vi "VSG25A_Main.vi"() -> ()   [LabVIEW 2014]
uses:
  Queue Control.ctl
  sg_lib/VSG25A.lvlib
panel:
  in  "RF On":bool
  in  "CW Button":bool
  in  "Sweep Button":bool
  in  "Ramp Button":bool
  in  "QAM Button":bool
  in  "FSK Button":bool
  in  "Multitone Button":bool
  in  "Pulse Button":bool
  in  "FM Button":bool
  in  "AM Button":bool
  in  "Amplitude (dBm)":dbl caption="Frequency"
  in  "Exit Button":bool caption="Blank Button"
  in  "Error In":errorcluster
  in  "Frequency":dbl
  in  "Connect Button":bool caption="Blank Button"
  out "Error Out":errorcluster
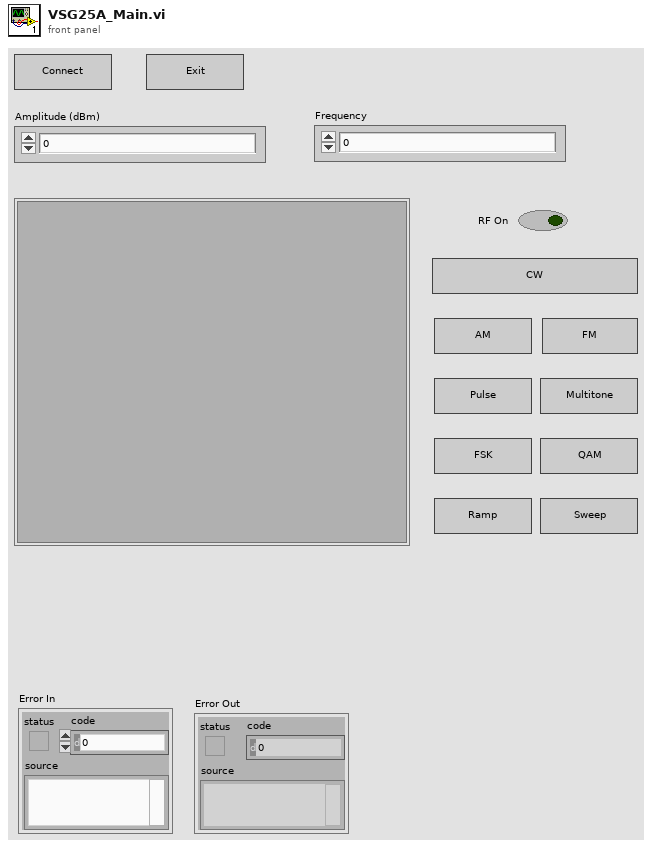
[diagram p1: front panel]
types:
  T1 = cluster{"Command":enum16{"Exit", "Connect"}, "Data":variant}
  T2 = typedef "Queue Control.ctl" = cluster{"Command":enum16{"Connect", "Exit", "RF On", "CW", "Sweep"}, "Data":variant}
  T3 = enum16{"Init", "Proc GUI Events", "Dispatch", "Exit"}
  T4 = enum16{"Connect", "Exit", "RF On", "CW", "Sweep"}
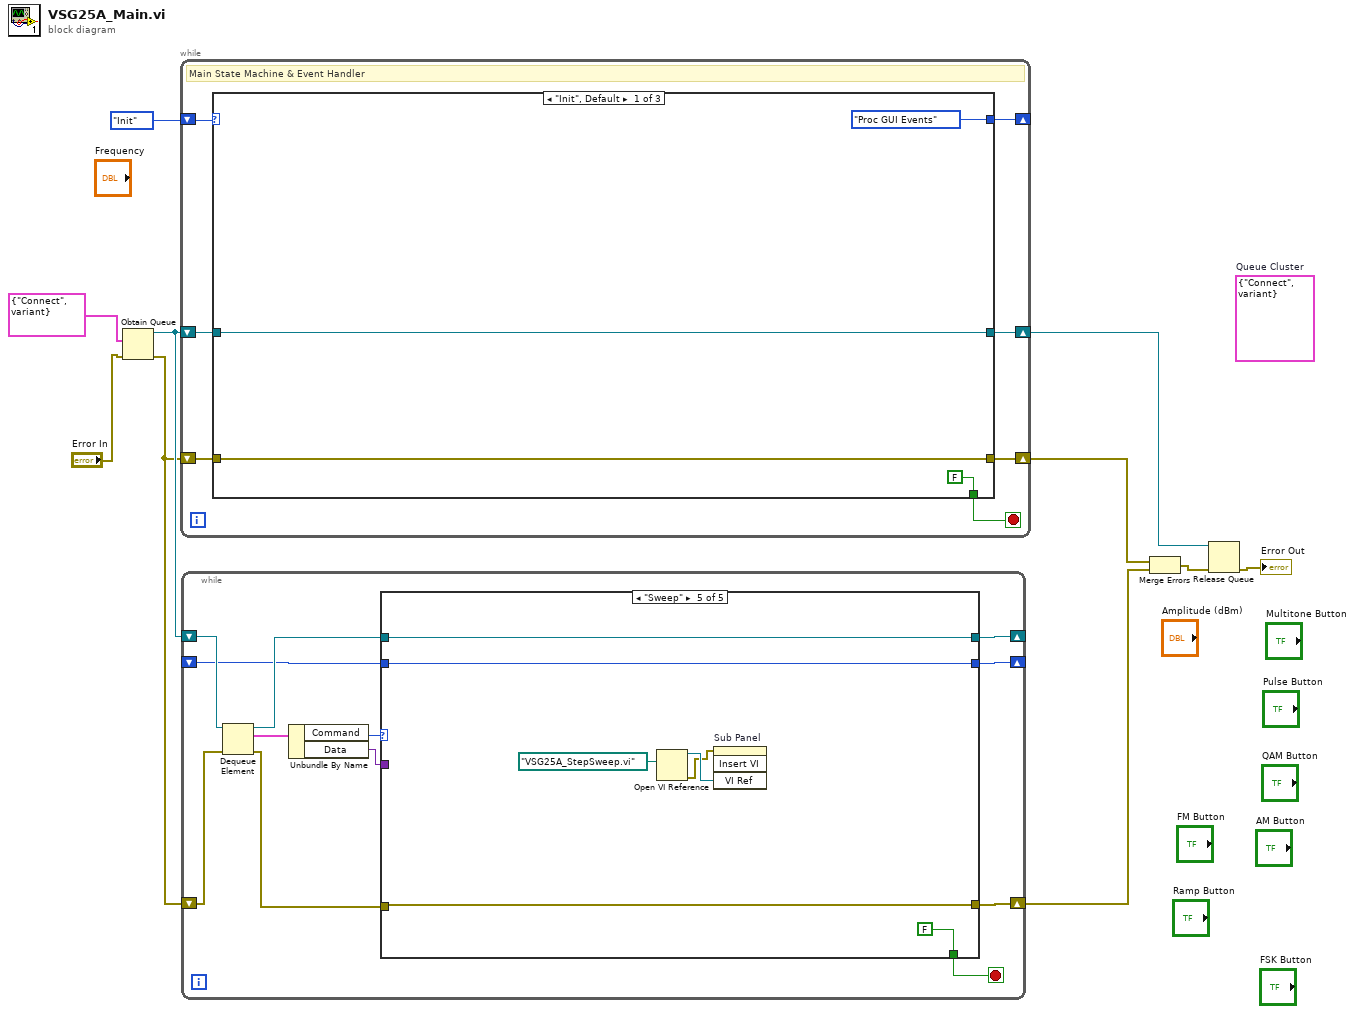
[diagram p0: block diagram]
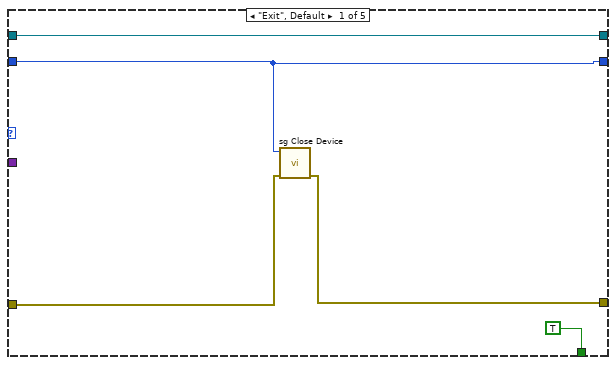
[diagram p2: hidden frame]
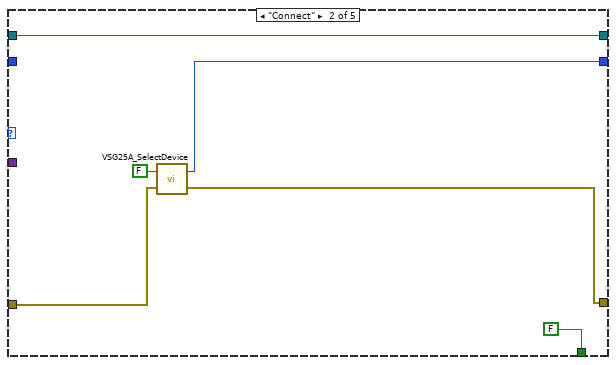
[diagram p3: hidden frame]
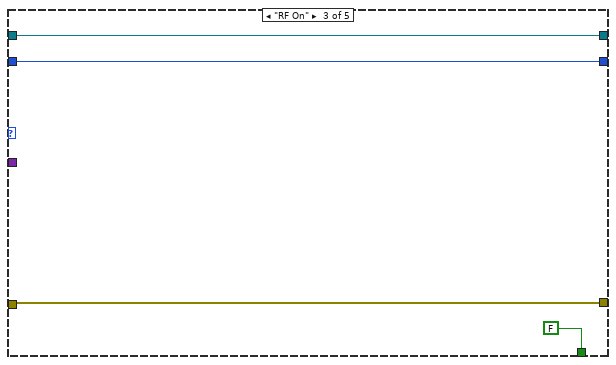
[diagram p4: hidden frame]
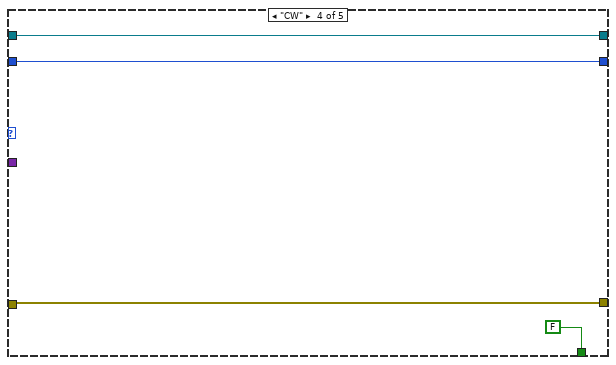
[diagram p5: hidden frame]
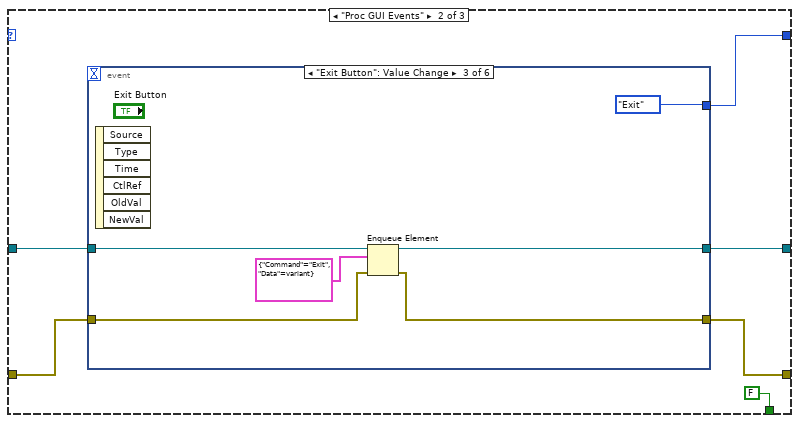
[diagram p6: hidden frame]
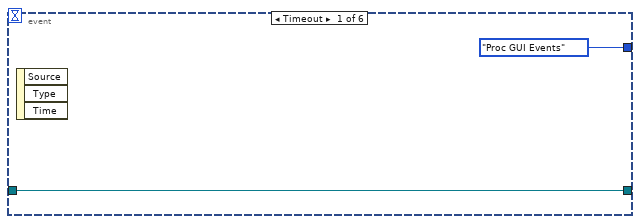
[diagram p7: hidden frame]
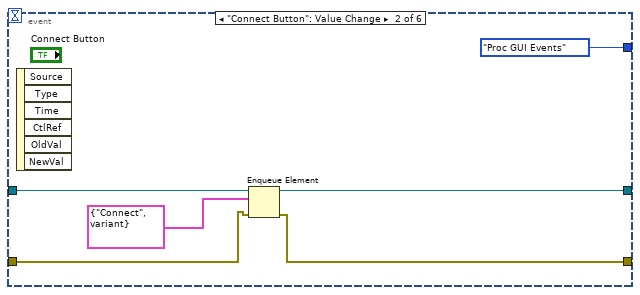
[diagram p8: hidden frame]
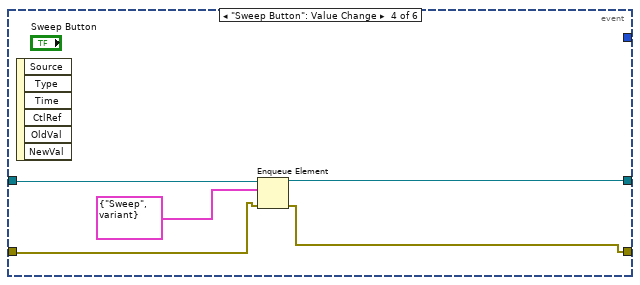
[diagram p9: hidden frame]
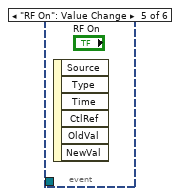
[diagram p10: hidden frame]
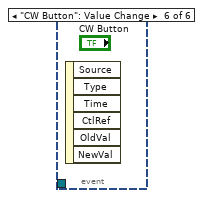
[diagram p11: hidden frame]
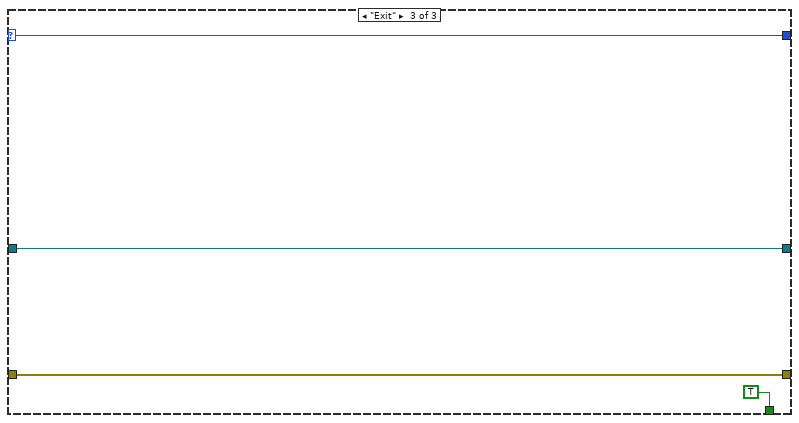
[diagram p12: hidden frame]
diagram:
  (unwired) T1 {"Command"=enum."Connect", "Data"=variant}  # Queue Cluster
  n1 = Obtain Queue(element data type=T2 {"Command"=enum."Connect", "Data"=variant} ("Queue Cluster"), error in (no error)="Error In") -> (queue out=w7:refnum<queue>, error out=w1:errorcluster)  [unwired: 3 in, 1 out]
  n2 = while {
    shift-right: [w14] -> _
    shift-left: T3."Init" -> [w17]
    shift-right: [w12] -> w3
    shift-left: w7 -> [w13]
    shift-right: [w11] -> w5
    shift-left: w1 -> [w16]
    stop <- w15 stop-if-true
    # "Main State Machine & Event Handler"
    n3 = case shown="\"Init\", Default" w17 {
      selector: w17 -> [_ _ w49]
      tunnel: w16 -> [w18 w23 w47]
      tunnel: [FALSE FALSE TRUE] -> w15
      tunnel: [T3."Proc GUI Events" w26 w49] -> w14
      tunnel: w13 -> [w19 w25 w48]
      tunnel: [w19 w24 w48] -> w12
      tunnel: [w18 w22 w47] -> w11
      frame "Init", Default {
      }
      frame "Proc GUI Events" {
        n4 = event shown="[2] \"Exit Button\": Value Change" {
          selector: _ -> [_ _ _ _ _ _]
          dyn-events: _ -> [_ _ _ _ _ _]
          timeout: _ -> [_ _ _ _ _ _]
          tunnel: [T3."Proc GUI Events" T3."Proc GUI Events" T3."Exit" _ _ _] -> w26
          tunnel: w25 -> [w28 w34 w40 w45 _ _]
          tunnel: [w28 w33 w39 w42 _ _] -> w24
          tunnel: w23 -> [_ w32 w38 w44 _ _]
          tunnel: [_ w31 w37 w43 _ _] -> w22
          event Timeout {
            n5 = event-data() -> ()  [unwired: 1 in, 3 out]
          }
          event "Connect Button": Value Change {
            n6 = event-data() -> ()  [unwired: 1 in, 6 out]
            n7 = Enqueue Element(queue=w34, element=T2 {"Command"=enum."Connect", "Data"=variant} ("Queue Cluster"), error in (no error)=w32) -> (queue out=w33:refnum<queue>, error out=w31:errorcluster)  [unwired: 1 in, 1 out]
          }
          event "Exit Button": Value Change {
            n8 = event-data() -> ()  [unwired: 1 in, 6 out]
            n9 = Enqueue Element(queue=w40, element=T2 {"Command"=enum."Exit", "Data"=variant}, error in (no error)=w38) -> (queue out=w39:refnum<queue>, error out=w37:errorcluster)  [unwired: 1 in, 1 out]
          }
          event "Sweep Button": Value Change {
            n10 = event-data() -> ()  [unwired: 1 in, 6 out]
            n11 = Enqueue Element(queue=w45, element=T2 {"Command"=enum."Sweep", "Data"=variant} ("Queue Cluster"), error in (no error)=w44) -> (queue out=w42:refnum<queue>, error out=w43:errorcluster)  [unwired: 1 in, 1 out]
          }
          event "RF On": Value Change {
            n12 = event-data() -> ()  [unwired: 1 in, 6 out]
          }
          event "CW Button": Value Change {
            n13 = event-data() -> ()  [unwired: 1 in, 6 out]
          }
        }
      }
      frame "Exit" {
      }
    }
  }
  n14 = while {
    shift-right: [w60] -> _
    shift-left: w7 -> [w62]
    shift-right: [w58] -> w6
    shift-left: w1 -> [w57]
    shift-right: [w54] -> _
    shift-left: _ -> [w53]
    stop <- w52 stop-if-true
    n15 = Dequeue Element(queue=w62, error in (no error)=w57) -> (queue out=w61:refnum<queue>, element=w56:T2, error out=w59:errorcluster)  [unwired: 1 in, 1 out]
    n16 = Unbundle By Name(w56) -> ("Command"=w55:T4, "Data"=w51:variant)
    n17 = case shown="\"Sweep\"" w55 {
      tunnel: w61 -> [w64 w73 w75 w79 w83]
      tunnel: [w64 w73 w75 w79 w83] -> w60
      tunnel: w59 -> [w66 w72 w74 w78 w82]
      tunnel: [w65 w68 w74 w78 w82] -> w58
      tunnel: [w67 w71 w76 w80 w84] -> w54
      tunnel: w53 -> [w67 _ w76 w80 w84]
      tunnel: [TRUE ("AutoSel") FALSE ("AutoSel") FALSE ("AutoSel") FALSE ("AutoSel") FALSE ("AutoSel")] -> w52
      tunnel: w51 -> [_ _ _ _ _]
      frame "Exit", Default {
        n18 = call "sg Close Device.vi"("error in (no error)"=w66, "device"=w67) -> ("error out"=w65:errorcluster)  [unwired: 8 in, 1 out]
      }
      frame "Connect" {
        n19 = call "VSG25A_SelectDevice.vi"("ErrorIn"=w72, "AutoSel"=FALSE) -> ("ErrorOut"=w68:errorcluster, "deviceHandle"=w71:i32)
      }
      frame "RF On" {
      }
      frame "CW" {
      }
      frame "Sweep" {
        n20 = Open VI Reference(vi path=path "VSG25A_StepSweep.vi") -> (vi reference=w87:refnum<vi>, error out=w86:errorcluster)  [unwired: 5 in]
        n21 = invoke on="Sub Panel" class="SubPanel" method="Insert VI"(error in=w86, "VI Ref"=w87) -> ()  [unwired: 2 in, 4 out]
      }
    }
  }
  n22 = Merge Errors(w5, w6) -> (w4:errorcluster)
  n23 = Release Queue(queue=w3, error in (no error)=w4) -> (error out=→"Error Out":errorcluster)  [unwired: 1 in, 2 out]
